vi "Read Plugin Type.vi"(8 "error in (no error)":errorcluster, 11 "Factory Plugin Framework in":refnum<class "Factory Plugin Framework.lvclass">=refnum) -> (0 "error out":errorcluster, 2 "Plugin Type":refnum<class>, 3 "Factory Plugin Framework out":refnum<class "Factory Plugin Framework.lvclass">)   [LabVIEW 2018, in "Factory Plugin Framework.lvlib" / "Factory Plugin Framework.lvclass"]
uses:
  Factory Plugin Framework.lvclass
  Factory Plugin Framework.lvclass/Factory Plugin Framework.ctl
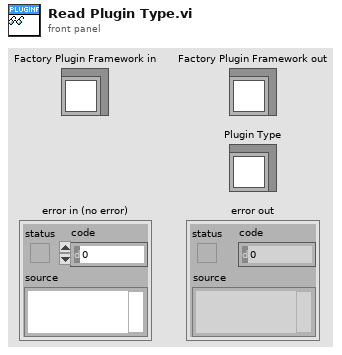
[diagram p1: front panel]
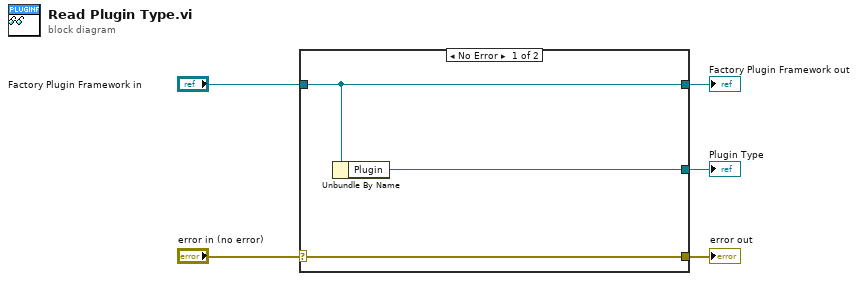
[diagram p0: block diagram]
diagram:
  n1 = case shown="No Error" "error in (no error)" {
    selector: "error in (no error)" -> [w8 w9]
    tunnel: [w8 w9] -> w4
    tunnel: [w7 w10] -> w2
    tunnel: "Factory Plugin Framework in" -> [w7 w10]
    tunnel: [w6 _] -> w1
    frame No Error {
      n2 = Unbundle By Name(w7) -> ("Plugin"=w6:refnum<class>)
    }
    frame Error {
    }
  }
  "error out" <- w4
  "Factory Plugin Framework out" <- w2
  "Plugin Type" <- w1
